vi "op_biti_v8.vi"() -> ()   [LabVIEW 2009]
panel:
  out "C=A OR B":dbl=251.0
  out "B":dbl=219.0
  out "A":dbl=107.0
  out "Array 5":bool[](array[boolean])=[TRUE, TRUE, TRUE, TRUE, TRUE, FALSE, TRUE, TRUE]
  in  "Array 4":bool[](array[boolean])=[TRUE, TRUE, FALSE, TRUE, TRUE, FALSE, TRUE, TRUE]
  out "Array 3":bool[](array[boolean])=[TRUE, TRUE, FALSE, TRUE, TRUE, FALSE, TRUE, TRUE]
  in  "Array 2":bool[](array[boolean])=[FALSE, TRUE, TRUE, FALSE, TRUE, FALSE, TRUE, TRUE]
  out "Array":bool[](array[boolean])=[FALSE, TRUE, TRUE, FALSE, TRUE, FALSE, TRUE, TRUE]
  # "A"
  # "B"
  # "C=A OR B"
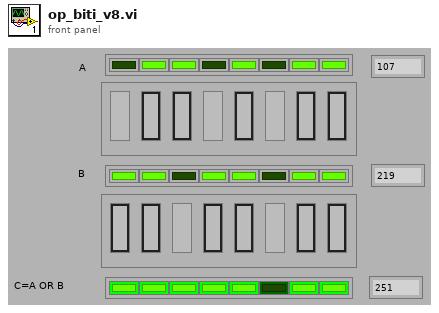
[diagram p1: front panel]
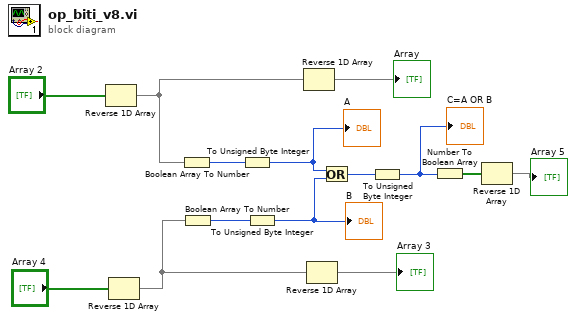
[diagram p0: block diagram]
diagram:
  n1 = Reverse 1D Array(array="Array 2") -> (reversed array=w13:bool[])
  n2 = Reverse 1D Array(array="Array 4") -> (reversed array=w10:bool[])
  n3 = Boolean Array To Number(Boolean array=w13) -> (number=w5:u32)
  n4 = Boolean Array To Number(Boolean array=w10) -> (number=w4:u32)
  n5 = To Unsigned Byte Integer(number=w5) -> (unsigned 8bit integer=w2:u8)
  "A" <- w2
  n6 = To Unsigned Byte Integer(number=w4) -> (unsigned 8bit integer=w1:u8)
  "B" <- w1
  n7 = Reverse 1D Array(array=w13) -> (reversed array=→"Array":bool[])
  n8 = Reverse 1D Array(array=w10) -> (reversed array=→"Array 3":bool[])
  n9 = Or(x=w2, y=w1) -> (x .or. y?=w6:u8)
  n10 = To Unsigned Byte Integer(number=w6) -> (unsigned 8bit integer=w3:u8)
  "C=A OR B" <- w3
  n11 = Number To Boolean Array(number=w3) -> (Boolean array=w8:bool[])
  n12 = Reverse 1D Array(array=w8) -> (reversed array=→"Array 5":bool[])
